vi "4461 - Create AO waveforms.vi"(6 "sampling info":cluster{"Fs":dbl, "#s":dbl}={"Fs"=1000.0, "#s"=1000.0} {"Fs" format="%.2p"}, 8 "error in (no error)":errorcluster, 10 "reset signal":bool, 11 "AO":T1={"AO amp (V)"=[0.1, 0.09, 0.08, 0.07, 0.06, 0.05, 0.04, 0.03], "AO DC (V)"=[0.0, 0.0, 0.0, 0.0, 0.0, 0.0, 0.0, 0.0], "AO f (Hz)"=[13.0, 13.0, 13.0, 13.0, 13.0, 13.0, 13.0, 13.0], "AO phi (°)"=[0.0, 0.0, 0.0, 0.0, 0.0, 0.0, 0.0, 0.0], "function"=[enum."Sine", enum."Sine", enum."Sine", enum."Sine", enum."Sine", enum."Sine", enum."Sine", enum."Sine"], "I+"=[]} {"AO f (Hz)" min=0.001 max=10000.0; "AO DC (V)" format="%.3p"; "AO amp (V)" format="%.3p"}) -> (0 "error out":errorcluster, 1 "phase out":dbl[](array[numeric]), 2 "AO Array":waveform(dbl)[](array[waveform]), 3 "AO out":T1={"AO amp (V)"=[0.1, 0.09, 0.08, 0.07, 0.06, 0.05, 0.04, 0.03], "AO DC (V)"=[0.0, 0.0, 0.0, 0.0, 0.0, 0.0, 0.0, 0.0], "AO f (Hz)"=[13.0, 13.0, 13.0, 13.0, 13.0, 13.0, 13.0, 13.0], "AO phi (°)"=[0.0, 0.0, 0.0, 0.0, 0.0, 0.0, 0.0, 0.0], "function"=[enum."Sine", enum."Sine", enum."Sine", enum."Sine", enum."Sine", enum."Sine", enum."Sine", enum."Sine"], "I+"=[]} {"AO f (Hz)" min=0.001 max=10000.0; "AO DC (V)" format="%.3p"; "AO amp (V)" format="%.3p"})   [LabVIEW 2016, in "LockinDAQ.lvclass"]
uses:
  LockinDAQ.lvclass
  Typedefs/AO-cluster.ctl
  Typedefs/AO_Amp-array.ctl
  Typedefs/AO_DC-array.ctl
  Typedefs/AO_f-array.ctl
  Typedefs/AO_phi-array.ctl
  Typedefs/Function-array.ctl
  Typedefs/Function-enum.ctl
  <vilib>/measure/NI_MABase.lvlib
panel:
  out "Waveform Chart":dbl[][](graph)
  out "Waveform Graph 2":waveform(dbl)[](graph)
  out "Numeric":i32
  # "1"
  # "2"
  # "3"
  # "4"
  # "5"
  # "6"
  # "7"
  # "8"
  # "1"
  # "2"
  # "3"
  # "4"
  # "5"
  # "6"
  # "7"
  # "8"
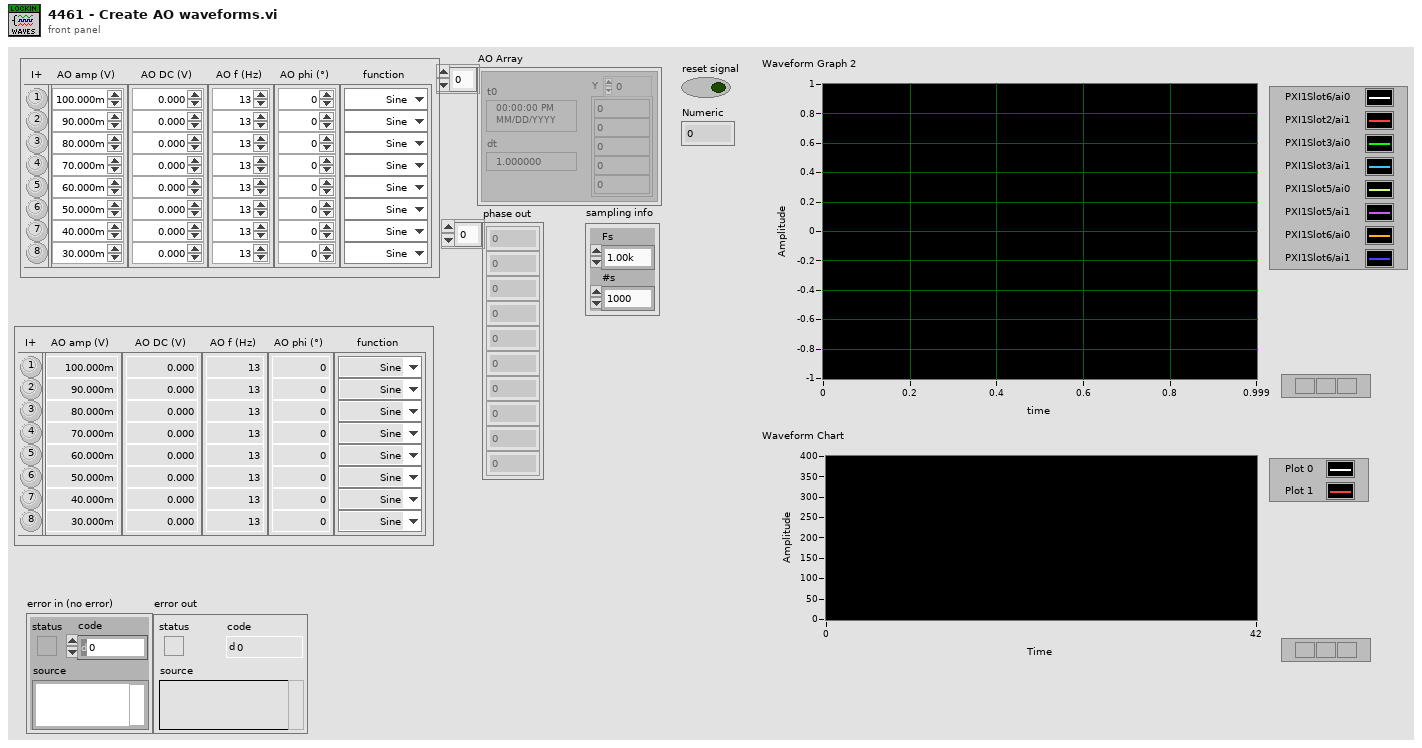
[diagram p1: front panel]
types:
  T1 = typedef "AO-cluster.ctl" = cluster{"AO amp (V)":T2, "AO DC (V)":T3, "AO f (Hz)":T4, "AO phi (°)":T5, "function":T6, "I+":bool[]}
  T2 = typedef "AO_Amp-array.ctl" = dbl[]
  T3 = typedef "AO_DC-array.ctl" = dbl[]
  T4 = typedef "AO_f-array.ctl" = dbl[]
  T5 = typedef "AO_phi-array.ctl" = dbl[]
  T6 = typedef "Function-array.ctl" = T7[]
  T7 = typedef "Function-enum.ctl" = enum16{"Sine", "Triangle", "Square", "Sawtooth"}
  T8 = enum16{"Sine Wave", "Triangle Wave", "Square Wave", "Sawtooth Wave"}
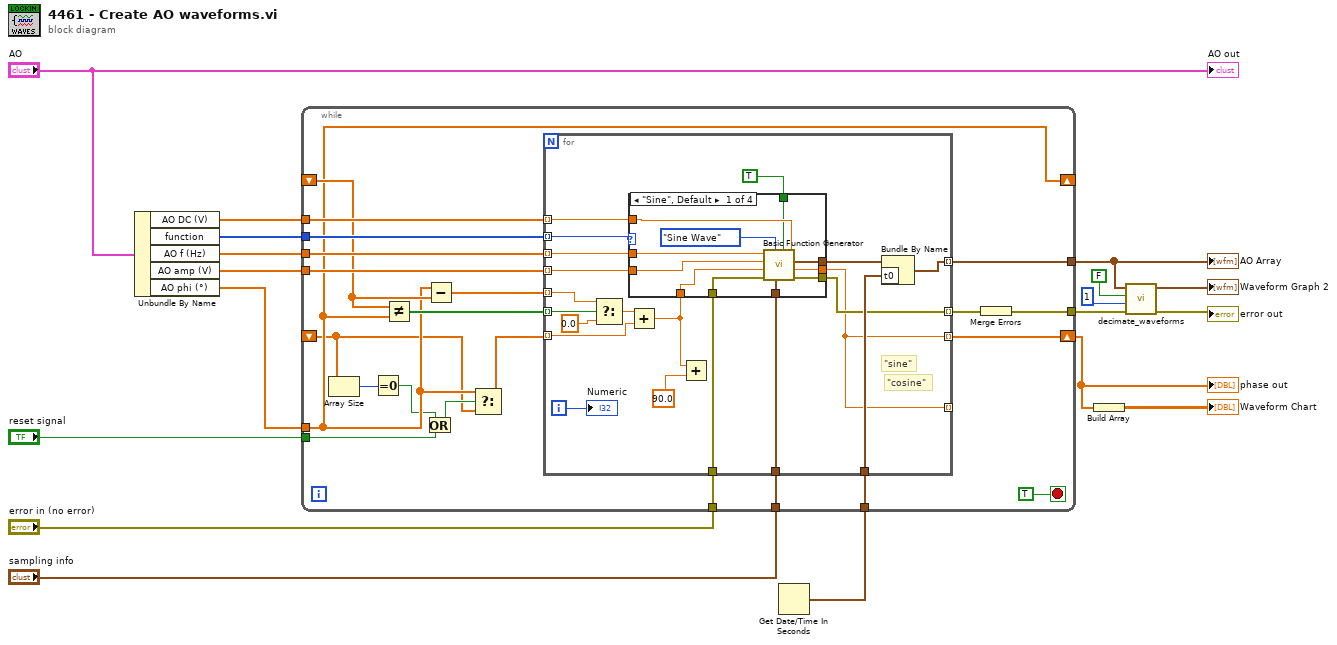
[diagram p0: block diagram]
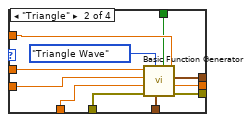
[diagram p2: hidden frame]
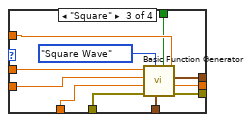
[diagram p3: hidden frame]
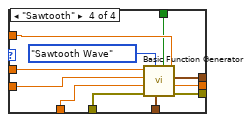
[diagram p4: hidden frame]
diagram:
  n1 = Unbundle By Name("AO") -> ("AO DC (V)"=w17:T3, "function"=w18:T6, "AO f (Hz)"=w14:T4, "AO amp (V)"=w15:T2, "AO phi (°)"=w3:T5)
  n2 = Get Date/Time In Seconds() -> (seconds since 1Jan1904=w1:timestamp)
  n3 = while {
    tunnel: w18 -> [w40]
    tunnel: w17 -> [w39]
    tunnel: "sampling info" -> [w38]
    tunnel: [w37] -> w12
    tunnel: w15 -> [w36]
    tunnel: w3 -> [w27]
    tunnel: w14 -> [w35]
    shift-right: [w27] -> _
    shift-left: _ -> [w32]
    shift-right: [w30] -> w6
    shift-left: _ -> [w19]
    tunnel: w1 -> [w29]
    tunnel: "reset signal" -> [w24]
    tunnel: "error in (no error)" -> [w22]
    tunnel: [w20] -> w9
    stop <- TRUE stop-if-true
    n4 = Array Size(array=w19) -> (size(s)=w28:i32)
    n5 = Equal To 0?(x=w28) -> (x = 0?=w25:bool)
    n6 = Not Equal?(x=w32, y=w27) -> (x != y?=w33:bool[])
    n7 = Or(x=w25, y=w24) -> (x .or. y?=w26:bool)
    n8 = Subtract(x=w27, y=w32) -> (x-y=w31:T5)
    n9 = Select(t=w27, s=w26, f=w19) -> (s? t:f=w23:T5)
    n10 = for {
      tunnel: w40 -> [w41] mode=indexing
      tunnel: w35 -> [w60] mode=indexing
      tunnel: w36 -> [w44] mode=indexing
      tunnel: w39 -> [w59] mode=indexing
      tunnel: [w49] -> w37 mode=indexing
      tunnel: w38 -> [w42]
      tunnel: w33 -> [w53] mode=indexing
      tunnel: w31 -> [w55] mode=indexing
      tunnel: [w46] -> w30 mode=indexing
      tunnel: w23 -> [w45] mode=indexing
      tunnel: w29 -> [w52]
      tunnel: [w46] -> _ mode=indexing
      tunnel: w22 -> [w48]
      tunnel: [w47] -> w21 mode=indexing
      i -> [w51]
      # "\"cosine\""
      # "\"sine\""
      n11 = Select(t=w55, s=w53, f=0.0) -> (s? t:f=w56:dbl)
      n12 = Add(x=w56, y=w45) -> (x+y=w43:dbl)
      n13 = case shown="\"Sine\", Default" w41 {
        tunnel: w60 -> [w71 w82 w93 w104]
        tunnel: w59 -> [w70 w81 w92 w103]
        tunnel: [w69 w80 w91 w102] -> w58
        tunnel: TRUE ("reset signal") -> [w68 w79 w90 w101]
        tunnel: w48 -> [w67 w78 w89 w100]
        tunnel: [w66 w77 w88 w99] -> w47
        tunnel: [w65 w76 w87 w98] -> w46
        tunnel: w44 -> [w64 w75 w86 w97]
        tunnel: w43 -> [w63 w74 w85 w96]
        tunnel: w42 -> [w62 w73 w84 w95]
        frame "Sine", Default {
          n14 = call <vilib>:"Basic Function Generator.vi"("offset"=w70, "reset signal"=w68, "sampling info"=w62, "signal type"=T8."Sine Wave", "error in (no error)"=w67, "phase"=w63, "amplitude"=w64, "frequency"=w71) -> ("error out"=w66:errorcluster, "phase out"=w65:dbl, "signal out"=w69:waveform(dbl))  [unwired: 1 in]
        }
        frame "Triangle" {
          n15 = call <vilib>:"Basic Function Generator.vi"("offset"=w81, "reset signal"=w79, "sampling info"=w73, "signal type"=T8."Triangle Wave", "error in (no error)"=w78, "phase"=w74, "amplitude"=w75, "frequency"=w82) -> ("error out"=w77:errorcluster, "phase out"=w76:dbl, "signal out"=w80:waveform(dbl))  [unwired: 1 in]
        }
        frame "Square" {
          n16 = call <vilib>:"Basic Function Generator.vi"("offset"=w92, "reset signal"=w90, "sampling info"=w84, "signal type"=T8."Square Wave", "error in (no error)"=w89, "phase"=w85, "amplitude"=w86, "frequency"=w93) -> ("error out"=w88:errorcluster, "phase out"=w87:dbl, "signal out"=w91:waveform(dbl))  [unwired: 1 in]
        }
        frame "Sawtooth" {
          n17 = call <vilib>:"Basic Function Generator.vi"("offset"=w103, "reset signal"=w101, "sampling info"=w95, "signal type"=T8."Sawtooth Wave", "error in (no error)"=w100, "phase"=w96, "amplitude"=w97, "frequency"=w104) -> ("error out"=w99:errorcluster, "phase out"=w98:dbl, "signal out"=w102:waveform(dbl))  [unwired: 1 in]
        }
      }
      n18 = Add(x=w43, y=90.0) -> ()  [unwired: 1 out]
      n19 = Bundle By Name(cluster=w58, "t0"=w52) -> (w49:waveform(dbl))
      "Numeric" <- w51
    }
    n20 = Merge Errors(w21) -> (w20:errorcluster)
  }
  "AO Array" <- w12
  "phase out" <- w6
  n21 = Build Array(w6) -> (→"Waveform Chart":dbl[][])
  n22 = call "decimate_waveforms.vi"("Input Signal"=w12, "averaging"=FALSE, "decimating factor"=1, "error in (no error)"=w9) -> ("Decimated Waveforms"=→"Waveform Graph 2":waveform(dbl)[], "error out"=→"error out":errorcluster)  [unwired: 5 in]
  "AO out" <- "AO"
